vi "Set LV Color.vi"(8 "error in (no error)":errorcluster, 10 "Color (black)":u32(colorbox), 11 "CMY Color.lvclass in":refnum<class "CMY Color.lvclass">) -> (0 "error out":errorcluster, 3 "CMY Color.lvclass out":refnum<class "CMY Color.lvclass">)   [LabVIEW 2020, in "CMY Color.lvclass"]
doc: "A method to set the color from a LabVIEW color value. If the same color cannot be shown in the color model, the closest color will be selected."
uses:
  CMY Color.lvclass
  CMY Color.lvclass/CMY Color.ctl
panel:
  # "expressionflow.com"
  # "Copyright (c) 2008 Tomi Maila. All rights reserved."
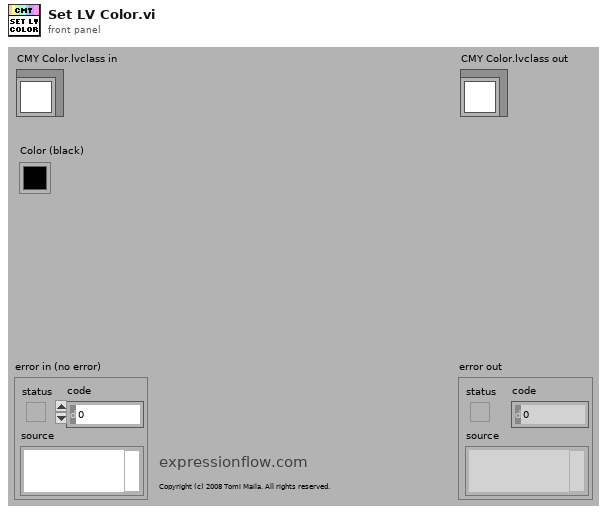
[diagram p1: front panel]
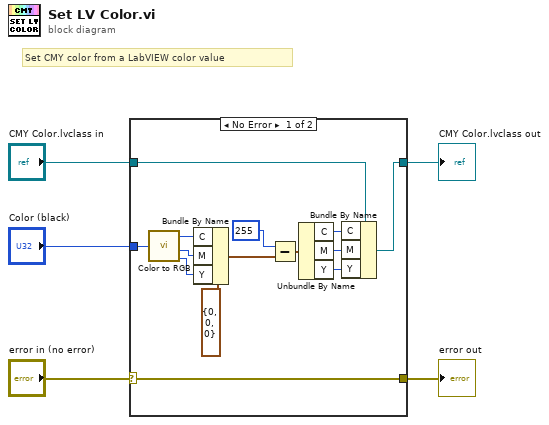
[diagram p0: block diagram]
diagram:
  # "Set CMY color from a LabVIEW color value"
  n1 = case shown="No Error" "error in (no error)" {
    selector: "error in (no error)" -> [w19 w20]
    tunnel: [w19 w20] -> w4
    tunnel: "CMY Color.lvclass in" -> [w18 w21]
    tunnel: [w17 w21] -> w2
    tunnel: "Color (black)" -> [w16 _]
    frame No Error {
      n2 = call <vilib>:"Color to RGB.vi"("Color"=w16) -> ("R"=w12:u8, "G"=w11:u8, "B"=w10:u8)  [unwired: 1 out]
      n3 = Bundle By Name(cluster=cluster{"C":u8, "M":u8, "Y":u8} {"C"=0, "M"=0, "Y"=0} ("RGB Value"), "C"=w12, "M"=w11, "Y"=w10) -> (w13:cluster{"C":u8, "M":u8, "Y":u8})
      n4 = Subtract(x=u8 255, y=w13) -> (x-y=w9:cluster{"C":u8, "M":u8, "Y":u8})
      n5 = Unbundle By Name(w9) -> ("C"=w8:u8, "M"=w7:u8, "Y"=w6:u8)
      n6 = Bundle By Name(cluster=w18, "C"=w8, "M"=w7, "Y"=w6) -> (w17:refnum<class "CMY Color.lvclass">)
    }
    frame Error {
    }
  }
  "error out" <- w4
  "CMY Color.lvclass out" <- w2
